vi "FRCts20_Backend_UpdateStartDate.vi"(6 "Message Attributes":T1, 8 "error in (no error)":errorcluster, 10 "Data":string, 11 "Engine_Refnums":T2) -> (0 "error out":errorcluster)   [LabVIEW 2013, in "FRCts20_Backend_Engine_Deprecated.lvlib"]
doc: "Configure competition information. Sets up competition dates."
uses:
  FRCts20_Backend_Engine_Deprecated.lvlib
  FRCts20_Backend_FGVDatesCommands.ctl
  FRCts20_Backend_Controls.lvlib
  <vilib>/Utility/config.llb/NI_LVConfig.lvlib
  <vilib>/Utility/config.llb/Write Key (String).vi
  Dependencies/Keyed Array/KeyedArray.ctl
  Dependencies/Keyed Array/Tools_KeyedArray.lvlib
  Dependencies/AMC/_SubVIs/TypeDefs/Message.ctl
  Dependencies/AMC/AMC.lvlib
  Dependencies/AMC/_SubVIs/TypeDefs/Message Queue.ctl
  FRCts20_Backend_EngineRefnums.ctl
  FRCts20_Backend_Engine.lvlib
  <vilib>/addons/database/Connection.llb/Conn ObjectReference.ctl
  <vilib>/addons/database/NI_Database_API.lvlib
  INI_Accessor/FRCts20_Backend_INI Controller.lvclass
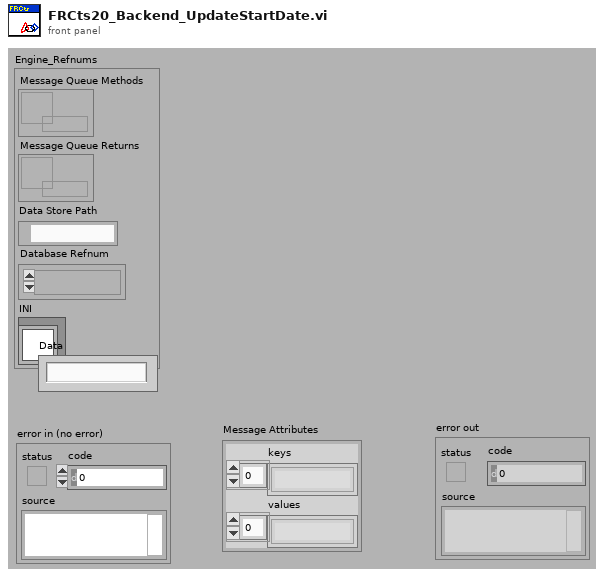
[diagram p1: front panel]
types:
  T1 = typedef "Tools_KeyedArray.lvlib/KeyedArray.ctl" = cluster{"keys":string[], "values":string[]}
  T2 = typedef "FRCts20_Backend_Engine.lvlib/FRCts20_Backend_EngineRefnums.ctl" = cluster{"Message Queue Methods":T3, "Message Queue Returns":T3, "Data Store Path":path, "Database Refnum":T4, "INI":refnum<class "FRCts20_Backend_INI Controller.lvclass">}
  T3 = typedef "AMC.lvlib/Message Queue.ctl" = refnum<queue>
  T4 = typedef "NI_Database_API.lvlib/Conn ObjectReference.ctl" = refnum<k1>
  T5 = typedef "FRCts20_Backend_Controls.lvlib/FRCts20_Backend_FGVDatesCommands.ctl" = enum16{"Set Dates", "Get Day", "Get First Day"}
  T6 = typedef "NI_LVConfig.lvlib/Config Data RefNum.ctl" = refnum<k1>
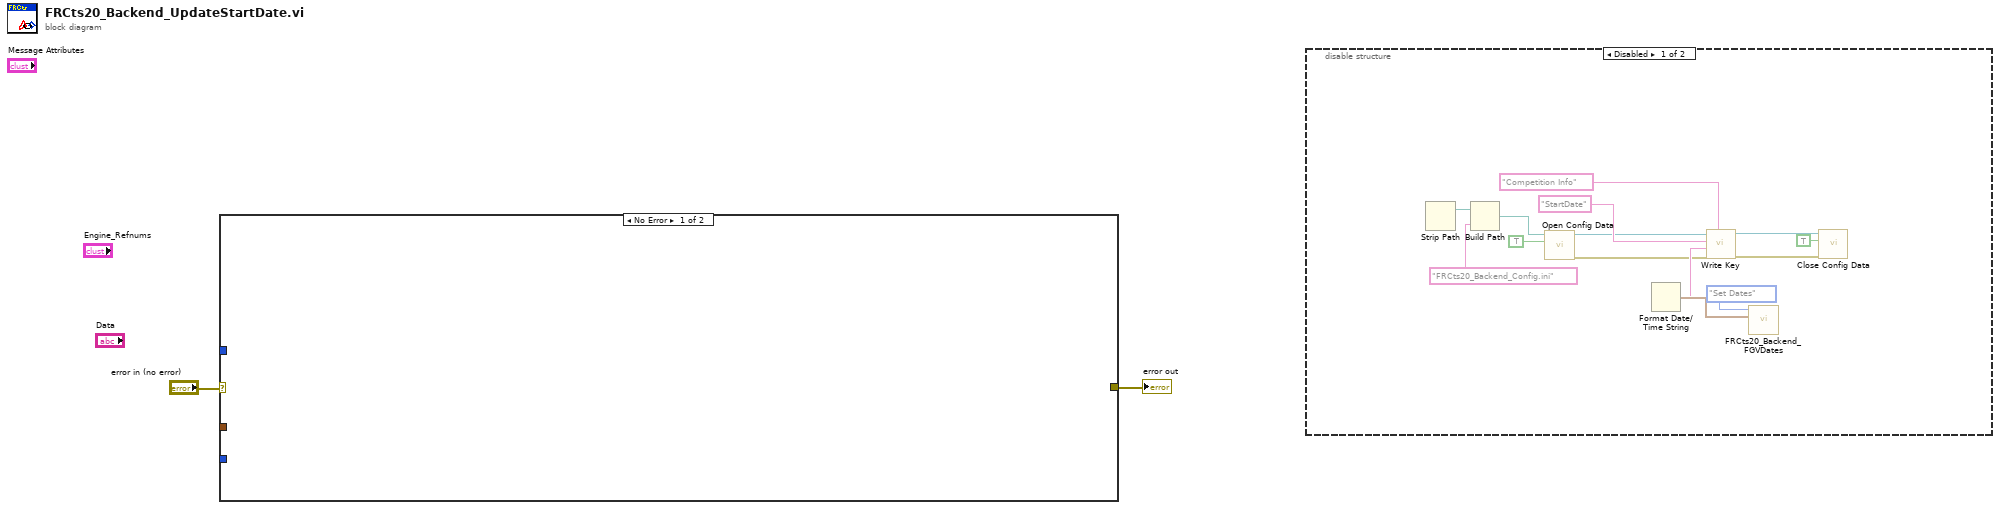
[diagram p0: block diagram]
diagram:
  n1 = case shown="No Error" "error in (no error)" {
    selector: "error in (no error)" -> [_ w6]
    tunnel: [_ w6] -> w4
    tunnel: [_ _] -> w3
    tunnel: [_ _] -> w2
    tunnel: [_ _] -> w1
    frame No Error {
    }
    frame Error {
    }
  }
  "error out" <- w4
  n2 = disable-structure shown="Disabled" {
    frame Disabled {
      n3 = Strip Path() -> (stripped path=w17:path)  [unwired: 1 in, 1 out]
      n4 = Build Path(base path=w17, name or relative path="FRCts20_Backend_Config.ini") -> (appended path=w19:path)
      n5 = call <vilib>:"Open Config Data.vi"("create file if necessary (T)"=TRUE, "configuration file path"=w19) -> ("error out"=w9:errorcluster, "refnum"=w10:T6, "error in (no error)"=w8:errorcluster)  [unwired: 6 in, 1 out]
      n6 = Format Date/Time String() -> (seconds (now)=w21:timestamp, date/time string=w20:string)  [unwired: 2 in]
      n7 = call-poly <vilib>:"Write Key.vi"("section"="Competition Info", "error in (no error)"=w9, "value"=w20, "key"="StartDate" ("section"), "refnum"=w10) -> ("error out"=w14:errorcluster, "refnum out"=w15:T6)  [unwired: 4 in, 1 out]
      n8 = call "FRCts20_Backend_FGVDates.vi"("Date"=w21, "Command"=FRCts20_Backend_FGVDatesCommands."Set Dates") -> ()  [unwired: 7 in, 3 out]
      n9 = call <vilib>:"Close Config Data.vi"("error in (no error)"=w14, "write file if changed (T)"=TRUE, "refnum"=w15) -> ()  [unwired: 7 in, 2 out]
    }
    frame Enabled {
    }
  }
